vi "SiosIfmSignalQuality.vi"(1 "Channel":i32(knob) scale=1.0..4.0, 2 "Signal select":i32(ring) items=["IFM_SIGNALQ_A1"=16, "IFM_SIGNALQ_O1"=32, "IFM_SIGNALQ_A2"=64, "IFM_SIGNALQ_O2"=128, "IFM_SIGNALQ_SUM"=256, "IFM_SIGNALQ_FREQ"=512, "IFM_SIGNALQ_STATE"=1024], 3 "Device Number":i32) -> (0 "Required Value":i32)   [LabVIEW 2009]
uses:
  siosifm.dll
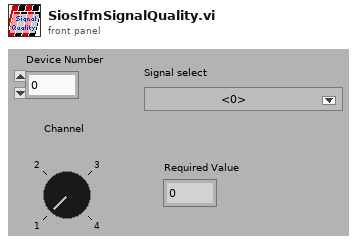
[diagram p1: front panel]
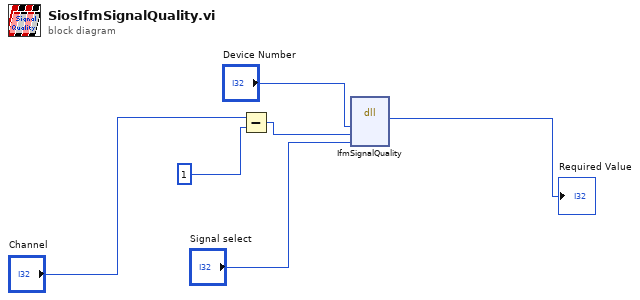
[diagram p0: block diagram]
diagram:
  n1 = Subtract(x="Channel", y=1) -> (x-y=w4:i32)
  n2 = dll-call lib="C:/WORK/Artem/RE-10/SIOS_IfmDLL/siosifm.dll" fn="IfmSignalQuality"("devNumber"="Device Number", "channel"=w4, "select"="Signal select") -> ("required value"=→"Required Value":i32)  [unwired: 6 in, 2 out]
